vi "Set.vi"(8 "error in":errorcluster, 9 "Sub Object":refnum<class "Sub Object.lvclass">, 10 "Sub Index":u8 format="%02x", 11 "Sub Objects Dictionary in":refnum<class "Sub Objects Dictionary.lvclass">) -> (0 "error out":errorcluster, 3 "Sub Objects Dictionary out":refnum<class "Sub Objects Dictionary.lvclass">)   [LabVIEW 2020, in "CANopen.lvlib" / "Sub Objects Dictionary.lvclass"]
doc: "Sets the Sub Object associated with the specified sub index. If the specified sub index is not found it creates a new Sub Object with the specified sub index."
uses:
  Sub Objects Dictionary.lvclass
  Sub Objects Dictionary.lvclass/Sub Objects Dictionary.ctl
  Sub Object/Sub Object.lvclass
  Ordered-Dictionary/Ordered Object Dictionary/Source/Ordered Object Dictionary.lvclass
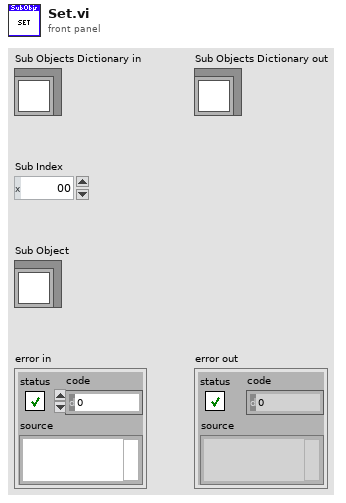
[diagram p1: front panel]
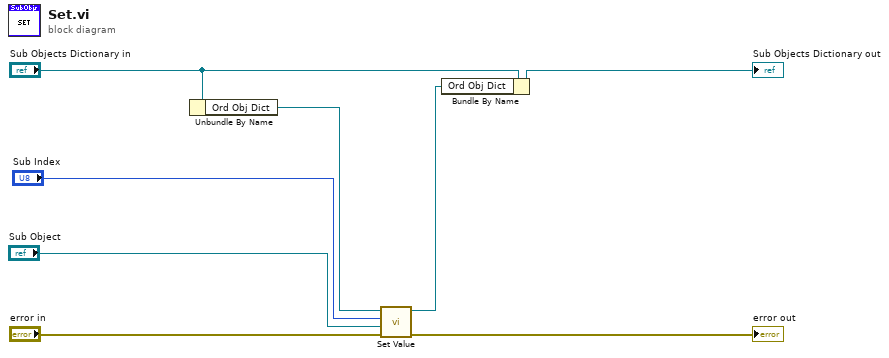
[diagram p0: block diagram]
diagram:
  n1 = Unbundle By Name("Sub Objects Dictionary in") -> ("Ord Obj Dict"=w5:refnum<class "Ordered Object Dictionary.lvclass">)
  n2 = call "Set Value.vi"("error in"="error in", "Value"="Sub Object", "Key"="Sub Index", "Ordered Object Dictionary in"=w5) -> ("error out"=→"error out":errorcluster, "Ordered Object Dictionary out"=w1:refnum<class "Ordered Object Dictionary.lvclass">)  [unwired: 6 in]
  n3 = Bundle By Name(cluster="Sub Objects Dictionary in", "Ord Obj Dict"=w1) -> (→"Sub Objects Dictionary out":refnum<class "Sub Objects Dictionary.lvclass">)
